vi "XY State Machine Example.vi"() -> ()   [LabVIEW 2019, in "xy_utilities.lvlib"]
uses:
  xy_utilities.lvlib
  subVIs/Derivative (single).vi
  subVIs/Get X and Y (multiple).vi
  subVIs/Add float (multiple).vi
  subVIs/Subtract float (multiple).vi
  subVIs/Multiply float (multiple).vi
  subVIs/Divide float (multiple).vi
  subVIs/Sort (multiple).vi
  subVIs/Swap X and Y (multiple).vi
  subVIs/Reverse (multiple).vi
  subVIs/Subset (multiple).vi
  subVIs/Interpolate (multiple).vi
  subVIs/FFT (multiple).vi
  subVIs/PS (multiple).vi
  subVIs/Resample (multiple).vi
panel:
  in  "Interval Units":enum16{"Points", "Data"}(ring)
  out "Differential":cluster{"X-array":dbl[], "Y-array":dbl[]}(graph)
  out "Processed States":string
  in  "y":dbl format="%#_6p"
  in  "x":dbl format="%#_6p"
  in  "Available States":i32(listbox) caption="States to Process"
  out "FFT":cluster{"f0":dbl, "df":dbl, "magnitude":dbl[]}[](graph)
  in  "Process Queue":string
  in  "PROCESS":bool
  in  "Configure":T1={"X Low"=0.05, "X High"=0.5, "X Step"=0.01, "Fake Point"=0.05} {"Fake Point" format="%#_6p"; "X Step" format="%#_6p"; "X High" format="%#_6p"; "X Low" format="%#_6p"}
  in  "Derivative Type":enum16{"dy/dx vs x", "dx/dy vs y"}(ring)
  in  "Interval":dbl=2.0
  out "Y Arrays":cluster{"Y-array":dbl[]}[](graph)
  out "X Arrays":cluster{"X-array":dbl[]}[](graph)
  in  "STOP":bool
  in  "Subset Slider":cluster{dbl, dbl}(slide)={0.75, 0.25} caption="Horizontal Slider" scale=0.0..1.0
  in  "Subset Method":enum16{"Slider (%)", "X[] min and max"}(ring)
  out "XY Data":cluster{"X-array":dbl[], "Y-array":dbl[]}[](graph)
  # "The \"Process Queue\" is a list of states that will execute when you press the \"PROCESS\" button. (XY: Load and UI: Display Data are added automatically to the beginning and end of the queue.)\n\nTo add states you can either:\n- Type directly into the Process Queue box.\nor:\n- Select a state in the \"Available States\" box that you want to add to the queue. ctl-v in the \"State Queue\" control to add to the queue.\n\nArguments for the various methods are found below"
  # "Arithmetic\n(+ - * /)"
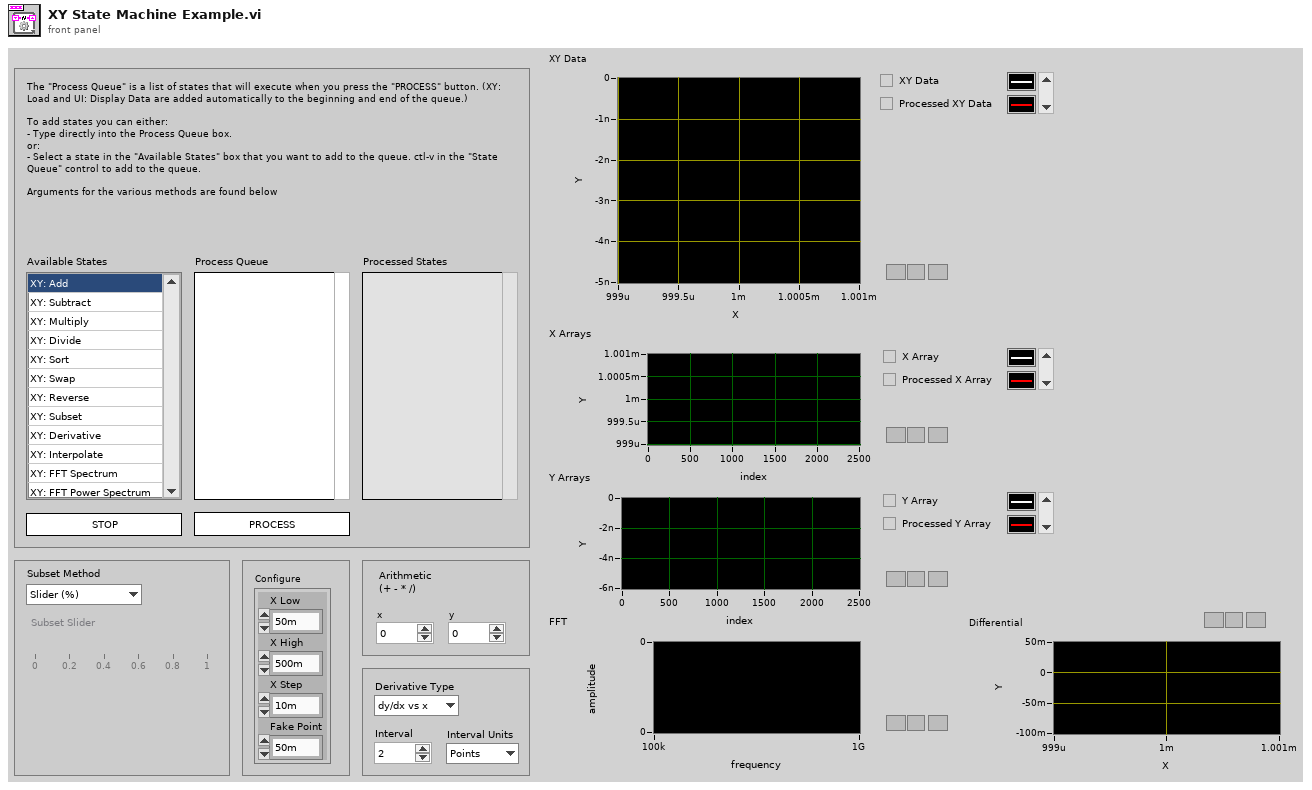
[diagram p1: front panel]
types:
  T1 = cluster{"X Low":dbl, "X High":dbl, "X Step":dbl, "Fake Point":dbl}
  T2 = enum32{"Invalid", "Standard", "Closed", "Hidden", "Minimized", "Maximized"}
  T3 = enum32{"invalid app kind", "Development System", "Run Time System", "Student Edition", "Embedded LabVIEW", "Evaluation", "Custom"}
  T4 = cluster{"Shift":bool, "Ctrl":bool, "Alt":bool, "Cmd":bool, "Opt":bool}
  T5 = cluster{"Core":cluster{"Current VI Reference":refnum<vi>, "Close Panel on Exit?":bool}, "XY Data (unprocessed)":cluster{"Intensity Data":dbl[], "Array":dbl[]}[], "XY Data":cluster{"Intensity Data":dbl[], "Array":dbl[]}[]}
  T6 = cluster{"Current VI Reference":refnum<vi>, "Close Panel on Exit?":bool}
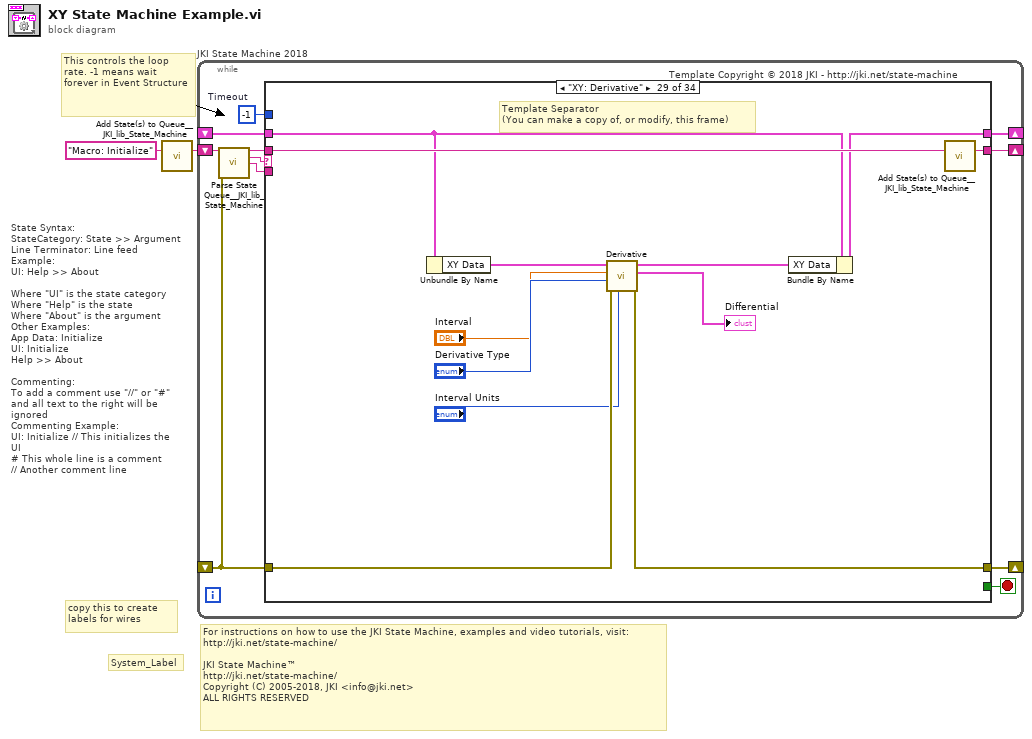
[diagram p0: block diagram]
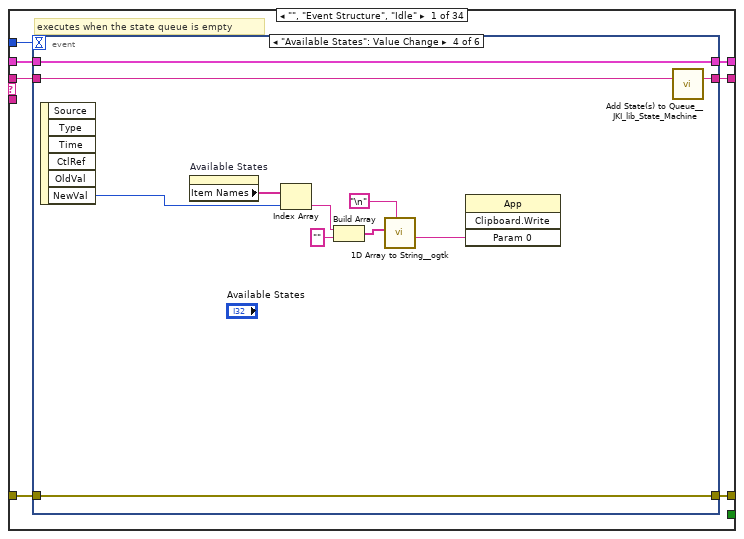
[diagram p2: hidden frame]
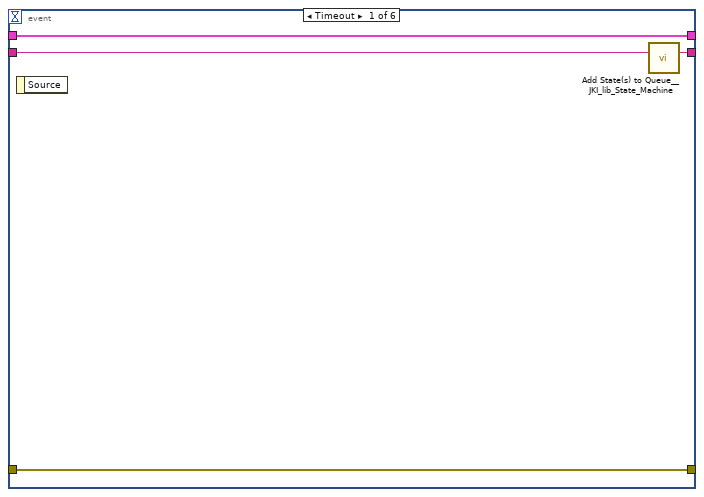
[diagram p3: hidden frame]
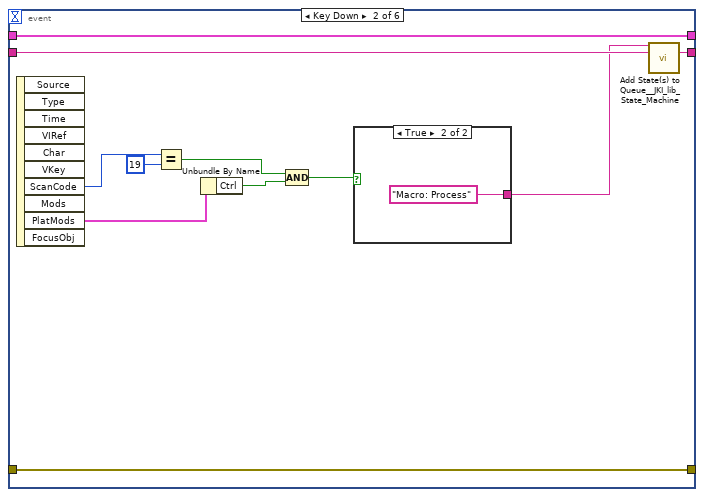
[diagram p4: hidden frame]
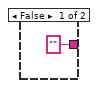
[diagram p5: hidden frame]
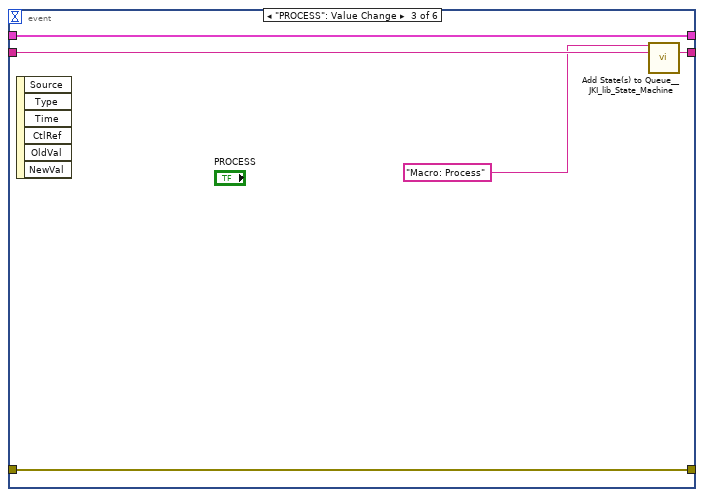
[diagram p6: hidden frame]
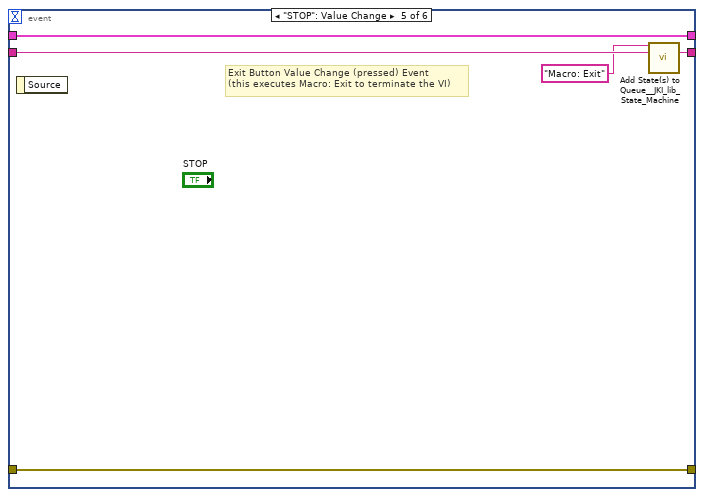
[diagram p7: hidden frame]
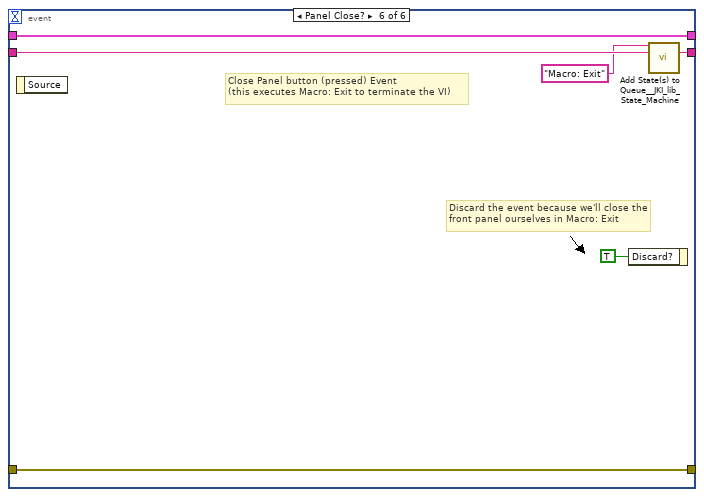
[diagram p8: hidden frame]
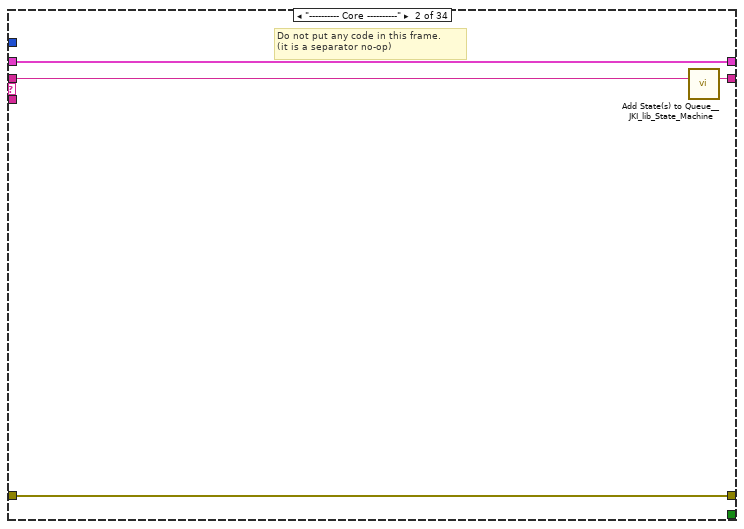
[diagram p9: hidden frame]
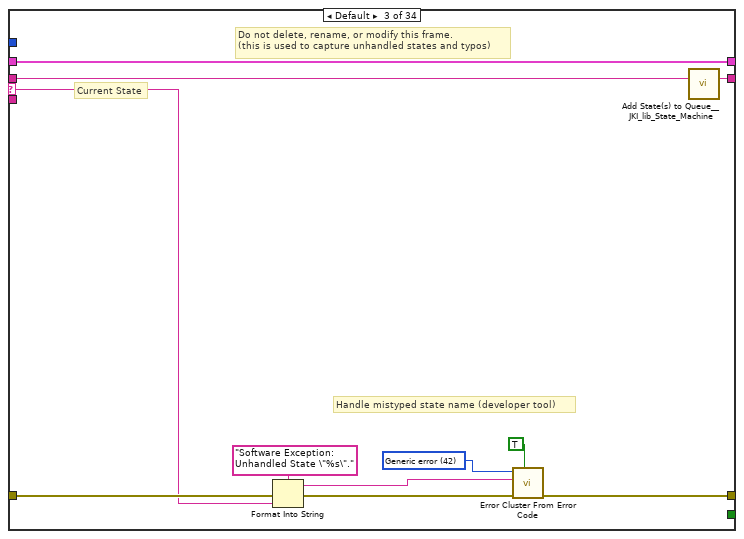
[diagram p10: hidden frame]
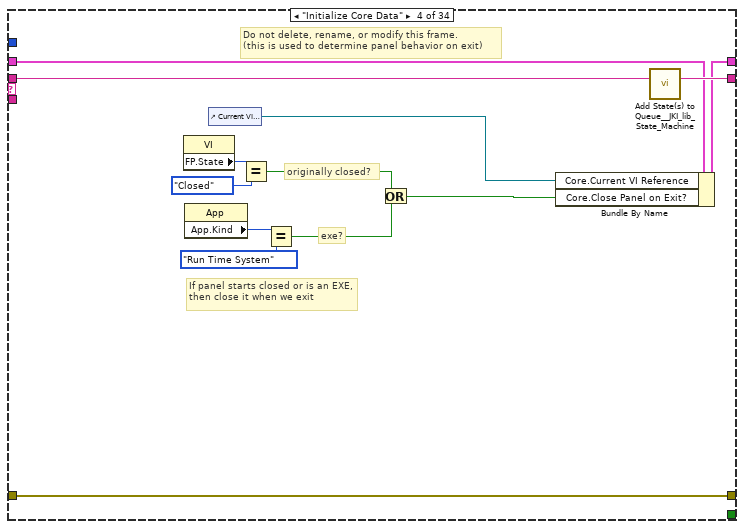
[diagram p11: hidden frame]
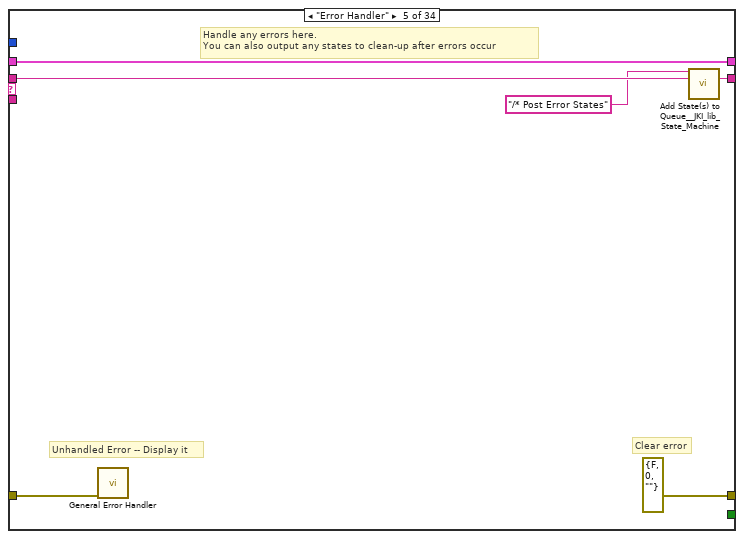
[diagram p12: hidden frame]
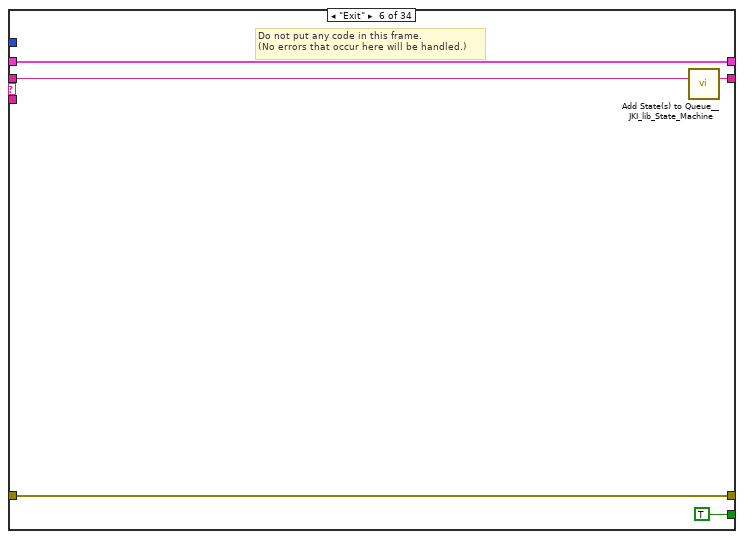
[diagram p13: hidden frame]
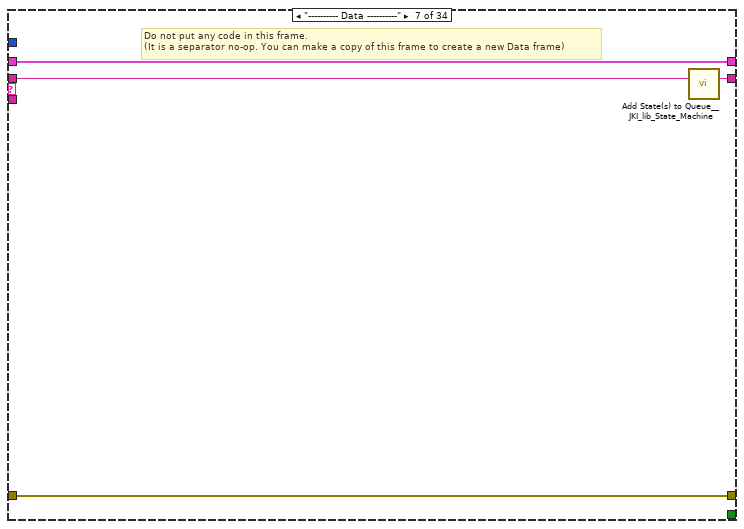
[diagram p14: hidden frame]
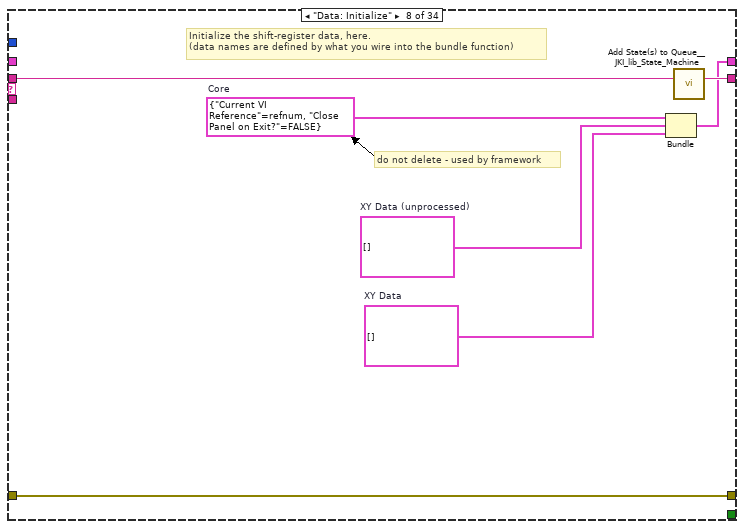
[diagram p15: hidden frame]
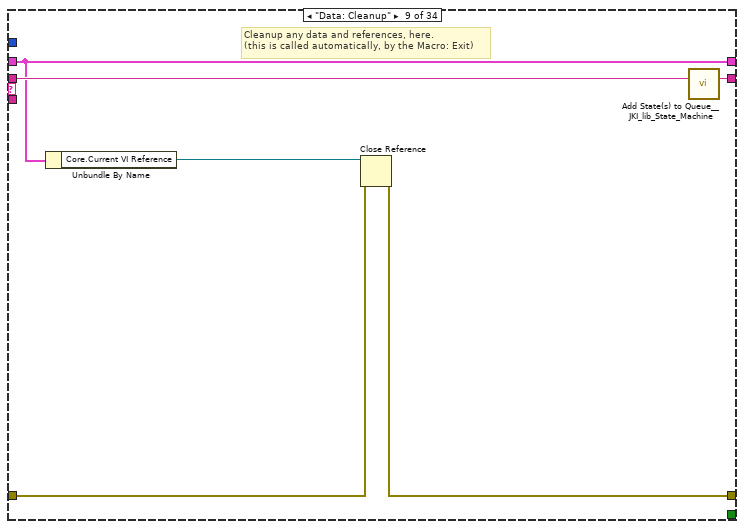
[diagram p16: hidden frame]
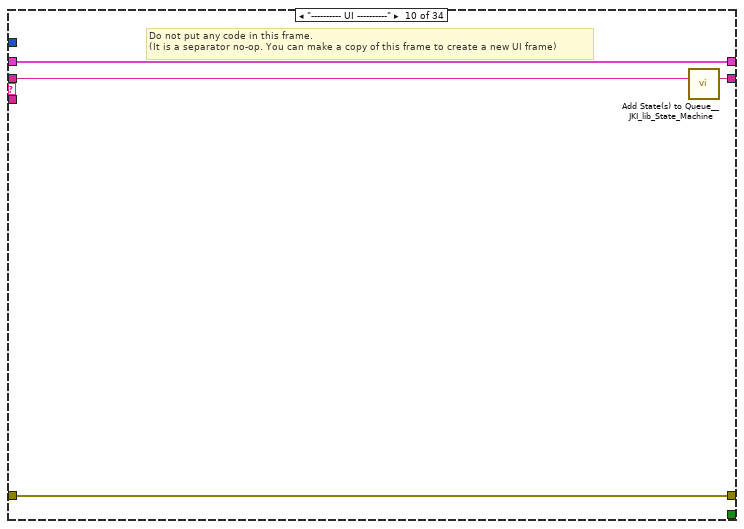
[diagram p17: hidden frame]
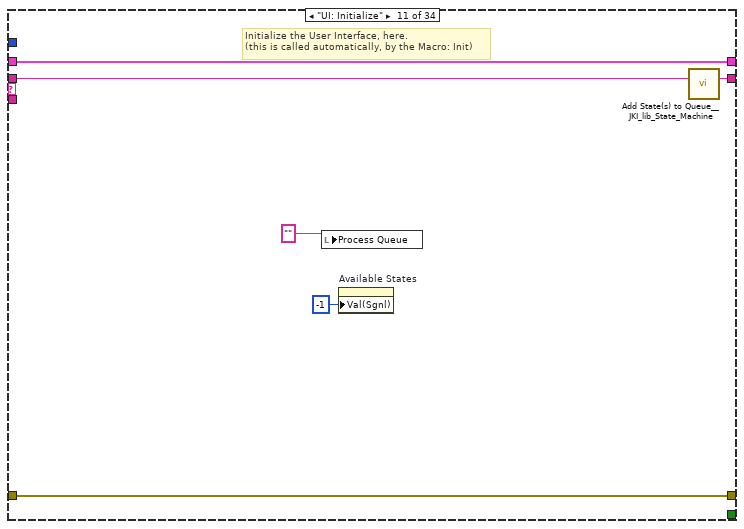
[diagram p18: hidden frame]
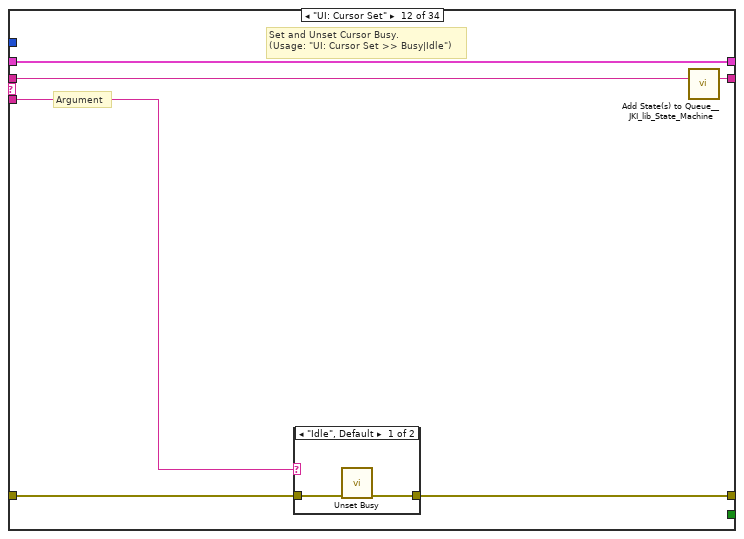
[diagram p19: hidden frame]
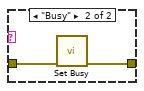
[diagram p20: hidden frame]
diagram:
  # "For instructions on how to use the JKI State Machine, examples and video tutorials, visit:\nhttp://jki.net/state-machine/\n\nJKI State Machine™\nhttp://jki.net/state-machine/\nCopyright (C) 2005-2018, JKI <info@jki.net>\nALL RIGHTS RESERVED"
  # "State Syntax:\nStateCategory: State >> Argument\nLine Terminator: Line feed\nExample:\nUI: Help >> About\n\nWhere \"UI\" is the state category\nWhere \"Help\" is the state\nWhere \"About\" is the argument\nOther Examples:\nApp Data: Initialize\nUI: Initialize\nHelp >> About\n\nCommenting:\nTo add a comment use \"//\" or \"#\" and all text to the right will be ignored\nCommenting Example:\nUI: Initialize // This initializes the UI\n# This whole line is a comment\n// Another comment line"
  # "copy this to create labels for wires"
  # "This controls the loop rate. -1 means wait forever in Event Structure"
  # "System_Label"
  n1 = call <vilib>:"Add State(s) to Queue__JKI_lib_State_Machine.vi"("State(s) in (\"\")"="Macro: Initialize") -> ("States Out"=w2:string)  [unwired: 14 in]
  n2 = while "JKI State Machine 2018" {
    shift-right: [w6] -> _
    shift-left: _ -> [w5]
    shift-right: [w9] -> _
    shift-left: _ -> [w3]
    shift-right: [w8] -> _
    shift-left: w2 -> [w10]
    stop <- w7 stop-if-true
    w4 = -1  # Timeout
    # "Template Copyright © 2018 JKI - http://jki.net/state-machine"
    n3 = call <vilib>:"Parse State Queue__JKI_lib_State_Machine.vi"("State Queue"=w10, "Error In (no error)"=w3) -> ("Remaining States"=w12:string, "Current State"=w13:string, "Arguments"=w11:string)  [unwired: 11 in]
    n4 = case shown="\"XY: Derivative\"" w13 {
      selector: w13 -> [_ _ w69 _ _ _ _ _ _ _ _ _ _ _ _ _ _ _ _ _ _ _ _ _ _ _ _ _ _ _ _ _ _ _]
      tunnel: w12 -> [w20 w68 w73 w92 w98 w103 w107 w114 w120 w124 w130 w136 w147 w223 w227 w232 w242 w250 w258 w264 w274 w284 w294 w304 w312 w320 w328 w338 w350 w359 w368 w377 w385 w393]
      tunnel: w11 -> [_ _ _ _ _ _ _ _ _ _ _ w131 w141 _ _ _ _ _ _ _ _ _ _ _ _ _ _ _ _ _ _ _ _ _]
      tunnel: w5 -> [w18 w65 w71 w85 w95 w101 w104 _ w115 w121 w128 w134 w143 w219 w224 w229 w239 w247 w255 w261 w271 w281 w291 w301 w309 w317 w325 w335 w347 w356 w365 w374 w382 w390]
      tunnel: [w17 w66 w75 w89 errorcluster {"status"=FALSE, "code"=0, "source"=""} ("error out") w100 w105 w111 w116 w122 w127 w132 w144 w216 w225 w230 w240 w248 w251 w262 w267 w277 w287 w297 w305 w313 w321 w331 w343 w352 w361 w371 w378 w386] -> w9
      tunnel: w3 -> [w16 w66 w74 w89 w94 w100 w105 w111 w117 w122 w127 w133 w145 w217 w225 w230 w240 w248 w252 w262 w268 w278 w288 w298 w306 w314 w322 w332 w344 w353 w362 w372 w379 w387]
      tunnel: [w19 w67 w72 w91 w97 w102 w106 w113 w119 w123 w129 w135 w146 w222 w226 w231 w241 w249 w257 w263 w273 w283 w293 w303 w311 w319 w327 w337 w349 w358 w367 w376 w384 w392] -> w8
      tunnel: [_ _ _ _ _ TRUE _ _ _ _ _ _ _ _ _ _ _ _ _ _ _ _ _ _ _ _ _ _ _ _ _ _ _ _] -> w7
      tunnel: [w15 w65 w71 w90 w95 w101 w104 w112 w115 w121 w128 w134 w143 w219 w224 w229 w239 w247 w254 w260 w270 w280 w290 w300 w308 w316 w324 w334 w346 w355 w364 w373 w381 w389] -> w6
      tunnel: w4 -> [w14 _ _ _ _ _ _ _ _ _ _ _ _ _ _ _ _ _ _ _ _ _ _ _ _ _ _ _ _ _ _ _ _ _]
      frame "", "Event Structure", "Idle" {
        # "executes when the state queue is empty"
        n5 = event shown="[3] \"Available States\": Value Change" {
          selector: _ -> [_ _ _ _ _ _]
          dyn-events: _ -> [_ _ _ _ _ _]
          timeout: w14 -> [_ _ _ _ _ _]
          tunnel: w20 -> [w24 w35 w42 w53 w58 w64]
          tunnel: [w23 w34 w41 w52 w57 w63] -> w19
          tunnel: w18 -> [w21 w32 w39 w50 w55 w61]
          tunnel: [w22 w33 w40 w51 w56 w62] -> w17
          tunnel: w16 -> [w22 w33 w40 w51 w56 w62]
          tunnel: [w21 w32 w39 w50 w55 w61] -> w15
          event Timeout {
            n6 = event-data() -> ()  [unwired: 1 in, 1 out]
            n7 = call <vilib>:"Add State(s) to Queue__JKI_lib_State_Machine.vi"("State(s) in (\"\")"=w24) -> ("States Out"=w23:string)  [unwired: 14 in]
          }
          event Key Down {
            n8 = event-data() -> ("ScanCode"=w25:i16, "PlatMods"=w26:T4)  [unwired: 1 in, 8 out]
            n9 = Equal?(x=w25, y=i16 19) -> (x = y?=w28:bool)
            n10 = Unbundle By Name(w26) -> ("Ctrl"=w29:bool)
            n11 = Compound Arithmetic op=AND(w28, w29) -> (w27:bool)
            n12 = case shown="True" w27 {
              tunnel: ["" ("State(s) in Front (\"\")") "Macro: Process" ("State(s) in Front (\"\")")] -> w30
              frame False {
              }
              frame True {
              }
            }
            n13 = call <vilib>:"Add State(s) to Queue__JKI_lib_State_Machine.vi"("State(s) in Front (\"\")"=w30, "State(s) in (\"\")"=w35) -> ("States Out"=w34:string)  [unwired: 13 in]
          }
          event "PROCESS": Value Change {
            n14 = event-data() -> ()  [unwired: 1 in, 6 out]
            n15 = call <vilib>:"Add State(s) to Queue__JKI_lib_State_Machine.vi"("State(s) in Front (\"\")"="Macro: Process" ("State(s) in Front (\"\")"), "State(s) in (\"\")"=w42) -> ("States Out"=w41:string)  [unwired: 13 in]
          }
          event "Available States": Value Change {
            n16 = event-data() -> ("NewVal"=w44:i32)  [unwired: 1 in, 5 out]
            n17 = property on="Available States" class="LstBox (strict)"() -> ("Item Names"=w45:string[])  [unwired: 2 in, 2 out]
            n18 = Index Array(array=w45, index=w44) -> (element=w49:string)
            n19 = Build Array(w49, "" ("element")) -> (w46:string[])
            n20 = call "1D Array to String__ogtk.vi"("delimiter (Tab)"="\n", "Array of Strings"=w46) -> ("delimited string"=w47:string)  [unwired: 9 in]
            n21 = invoke class="App" method="Clipboard.Write"("Param 0"=w47) -> ()  [unwired: 3 in, 4 out]
            n22 = call <vilib>:"Add State(s) to Queue__JKI_lib_State_Machine.vi"("State(s) in (\"\")"=w53) -> ("States Out"=w52:string)  [unwired: 14 in]
          }
          event "STOP": Value Change {
            # "Exit Button Value Change (pressed) Event\n(this executes Macro: Exit to terminate the VI)"
            n23 = event-data() -> ()  [unwired: 1 in, 1 out]
            n24 = call <vilib>:"Add State(s) to Queue__JKI_lib_State_Machine.vi"("State(s) in Front (\"\")"="Macro: Exit", "State(s) in (\"\")"=w58) -> ("States Out"=w57:string)  [unwired: 13 in]
          }
          event Panel Close? {
            # "Discard the event because we'll close the front panel ourselves in Macro: Exit"
            # "Close Panel button (pressed) Event\n(this executes Macro: Exit to terminate the VI)"
            n25 = event-data() -> ()  [unwired: 1 in, 1 out]
            n26 = event-data("Discard?"=TRUE) -> ()  [unwired: 1 in, 1 out]
            n27 = call <vilib>:"Add State(s) to Queue__JKI_lib_State_Machine.vi"("State(s) in Front (\"\")"="Macro: Exit", "State(s) in (\"\")"=w64) -> ("States Out"=w63:string)  [unwired: 13 in]
          }
        }
      }
      frame "---------- Core ----------" {
        # "Do not put any code in this frame.\n(it is a separator no-op)"
        n28 = call <vilib>:"Add State(s) to Queue__JKI_lib_State_Machine.vi"("State(s) in (\"\")"=w68) -> ("States Out"=w67:string)  [unwired: 14 in]
      }
      frame Default {
        w78 = 42 items=["No error", "Argument error", "Memory is full", "Out of zone", "End of file", "File already open", "Generic file I/O error", "File not found", "File permission error", "Disk is full", "Duplicate path", "Too many files open", "System feature not enabled", "Resource file not found", "Cannot add resource", "Resource not found", "Image not found", "Image memory error", "Pen does not exist", "Config type invalid", "Config token not found", "Config parse error", "Config memory error", "Bad external code format", "Bad external code offset", "External code not present", "Null window", "Destroy window error", "Null menu", "Print aborted", "Bad print record", "Print driver error", "Windows error during printing", "Memory error during printing", "Print dialog error", "Generic print error", "Invalid device refnum", "Device not found", "Device parameter error", "Device unit error", "Cannot open device", "Device call aborted", "Generic error", "Cancelled by user", "Object ID too low", "Object ID too high", "Object not in heap", "Unknown heap", "Unknown object (invalid DefProc)", "Unknown object (DefProc not in table)", "Message out of range", "Invalid (null) method", "Unknown message", "Manager call not supported", "Bad address", "Network operation in progress", "Network operation timed out", "Connection is busy", "Network attribute not supported", "Network error", "Address in use", "System out of memory", "Connection aborted", "Connection refused", "Not connected", "Already connected", "Connection closed", "Initialization error (interapplication manager)", "Bad occurrence", "Wait on unbound occurrence handler", "Occurrence queue overflow", "Datalog type conflict", "Unused", "Unrecognized type (interapplication manager)", "Memory corrupt", "Failed to make temporary DLL", "Old CIN version", "Drag socket not found", "Failed to load drop-object", "Failed to register OLE object", "Failed to release OLE object", "Format specifier type mismatch", "Unknown format specifier", "Too few format specifiers", "Too many format specifiers", "Scan failed", "Newer CIN version", "Error converting to variant", "Runtime menu error", "Password tampered", "Variant attribute not found", "Incompatible variant data type", "Event data is not available", "Event Store is not present", "Occurrence is not found", "Event Queue is not created", "Event info is not available", "Refnum passed is NULL", "Error retrieving Class GUID", "Error retrieving CoClass GUID", "Error retrieving TypeLib GUID.", "Bad built application magic bytes.", "Specific driver is different from the specific driver associated with the Logical Name.", "There is no session opened to the class driver.", "Max Error", "MAX - Error with config objects", "MAX - Error loading configuration", "MAX - Group not supported"]
        # "Current State"
        # "Do not delete, rename, or modify this frame.\n(this is used to capture unhandled states and typos)"
        # "Handle mistyped state name (developer tool)"
        n29 = Format Into String(format string="Software Exception: Unhandled State \"%s\"." ("message"), error in=w74, w69) -> (resulting string=w77:string, error out=w76:errorcluster)  [unwired: 1 in]
        n30 = call <vilib>:"Error Cluster From Error Code.vi"("show call chain? (False)"=TRUE, "error in (no error)"=w76, "error message (\"\")"=w77, "error code (0)"=w78) -> ("error out"=w75:errorcluster)  [unwired: 5 in]
        n31 = call <vilib>:"Add State(s) to Queue__JKI_lib_State_Machine.vi"("State(s) in (\"\")"=w73) -> ("States Out"=w72:string)  [unwired: 14 in]
      }
      frame "Initialize Core Data" {
        # "Do not delete, rename, or modify this frame.\n(this is used to determine panel behavior on exit)"
        # "originally closed?"
        # "exe?"
        # "If panel starts closed or is an EXE, then close it when we exit"
        n32 = property class="VI"() -> ("FP.State"=w82:T2)  [unwired: 2 in, 2 out]
        n33 = property class="App"() -> ("App.Kind"=w88:T3)  [unwired: 2 in, 2 out]
        n34 = control-ref of="Current VI Reference"() -> (w83:refnum<vi>)
        n35 = Equal?(x=w82, y=T2."Closed" ("Front Panel Window:State")) -> (x = y?=w80:bool)
        n36 = Equal?(x=w88, y=T3."Run Time System" ("Application:Kind")) -> (x = y?=w86:bool)
        n37 = Or(x=w80, y=w86) -> (x .or. y?=w84:bool)
        n38 = Bundle By Name(cluster=w85, "Core.Current VI Reference"=w83, "Core.Close Panel on Exit?"=w84) -> (w90:T5)
        n39 = call <vilib>:"Add State(s) to Queue__JKI_lib_State_Machine.vi"("State(s) in (\"\")"=w92) -> ("States Out"=w91:string)  [unwired: 14 in]
      }
      frame "Error Handler" {
        # "Unhandled Error -- Display it"
        # "Handle any errors here.\nYou can also output any states to clean-up after errors occur"
        # "Clear error"
        n40 = call <vilib>:"General Error Handler.vi"("error in (no error)"=w94) -> ()  [unwired: 10 in, 5 out]
        n41 = call <vilib>:"Add State(s) to Queue__JKI_lib_State_Machine.vi"("State(s) in Front (\"\")"="/* Post Error States", "State(s) in (\"\")"=w98) -> ("States Out"=w97:string)  [unwired: 13 in]
      }
      frame "Exit" {
        # "Do not put any code in this frame.\n(No errors that occur here will be handled.)"
        n42 = call <vilib>:"Add State(s) to Queue__JKI_lib_State_Machine.vi"("State(s) in (\"\")"=w103) -> ("States Out"=w102:string)  [unwired: 14 in]
      }
      frame "---------- Data ----------" {
        # "Do not put any code in this frame.\n(It is a separator no-op. You can make a copy of this frame to create a new Data frame)"
        n43 = call <vilib>:"Add State(s) to Queue__JKI_lib_State_Machine.vi"("State(s) in (\"\")"=w107) -> ("States Out"=w106:string)  [unwired: 14 in]
      }
      frame "Data: Initialize" {
        w108 = cluster{"Intensity Data":dbl[], "Array":dbl[]}[] []  # XY Data
        w109 = cluster{"Intensity Data":dbl[], "Array":dbl[]}[] []  # XY Data (unprocessed)
        w110 = T6 {"Current VI Reference"=refnum, "Close Panel on Exit?"=FALSE}  # Core
        # "do not delete - used by framework"
        # "Initialize the shift-register data, here.\n(data names are defined by what you wire into the bundle function)"
        n44 = Bundle("Core"=w110, "XY Data (unprocessed)"=w109, "XY Data"=w108) -> (w112:T5)  [unwired: 1 in]
        n45 = call <vilib>:"Add State(s) to Queue__JKI_lib_State_Machine.vi"("State(s) in (\"\")"=w114) -> ("States Out"=w113:string)  [unwired: 14 in]
      }
      frame "Data: Cleanup" {
        # "Cleanup any data and references, here.\n(this is called automatically, by the Macro: Exit)"
        n46 = Unbundle By Name(w115) -> ("Core.Current VI Reference"=w118:refnum<vi>)
        n47 = Close Reference(reference=w118, error in (no error)=w117) -> (error out=w116:errorcluster)
        n48 = call <vilib>:"Add State(s) to Queue__JKI_lib_State_Machine.vi"("State(s) in (\"\")"=w120) -> ("States Out"=w119:string)  [unwired: 14 in]
      }
      frame "---------- UI ----------" {
        # "Do not put any code in this frame.\n(It is a separator no-op. You can make a copy of this frame to create a new UI frame)"
        n49 = call <vilib>:"Add State(s) to Queue__JKI_lib_State_Machine.vi"("State(s) in (\"\")"=w124) -> ("States Out"=w123:string)  [unwired: 14 in]
      }
      frame "UI: Initialize" {
        # "Initialize the User Interface, here.\n(this is called automatically, by the Macro: Init)"
        n50 = local write "Process Queue"("" ("Process States")) -> ()
        n51 = property on="Available States" class="LstBox (strict)"("Val(Sgnl)"=-1 ("Value (Signaling)")) -> ()  [unwired: 2 in, 2 out]
        n52 = call <vilib>:"Add State(s) to Queue__JKI_lib_State_Machine.vi"("State(s) in (\"\")"=w130) -> ("States Out"=w129:string)  [unwired: 14 in]
      }
      frame "UI: Cursor Set" {
        # "Argument"
        # "Set and Unset Cursor Busy.\n(Usage: \"UI: Cursor Set >> Busy|Idle\")"
        n53 = case shown="\"Idle\", Default" w131 {
          tunnel: w133 -> [w138 w140]
          tunnel: [w137 w139] -> w132
          frame "Idle", Default {
            n54 = call <vilib>:"Unset Busy.vi"("error in (no error)"=w138) -> ("error out"=w137:errorcluster)  [unwired: 10 in]
          }
          frame "Busy" {
            n55 = call <vilib>:"Set Busy.vi"("error in (no error)"=w140) -> ("error out"=w139:errorcluster)  [unwired: 9 in, 1 out]
          }
        }
        n56 = call <vilib>:"Add State(s) to Queue__JKI_lib_State_Machine.vi"("State(s) in (\"\")"=w136) -> ("States Out"=w135:string)  [unwired: 14 in]
      }
      frame "UI: Front Panel State" {
        # "Argument"
        # "Set Front Panel Open or Closed\n(Usage: \"UI: Front Panel State >> Open|Close\")"
        n57 = Unbundle By Name(w143) -> ("Core.Current VI Reference"=w142:refnum<vi>)
        n58 = case shown="\"Maximize\", \"Maximized\"" w141 {
          tunnel: w145 -> [w153 w168 w179 w192 w205]
          tunnel: [w155 w169 w181 w194 w207] -> w144
          tunnel: w142 -> [w154 w166 w180 w193 w206]
          frame "Open", "Standard", Default {
            w148 = T2."Standard" ("State")
            n59 = property class="VI"(reference=w154, error in=w153) -> (reference out=w151:refnum<vi>, error out=w152:errorcluster, "FP.State"=w150:T2)
            n60 = Not Equal?(x=w150, y=w148) -> (x != y?=w149:bool)
            n61 = case shown="True" w149 {
              tunnel: [w159 w161] -> w155
              tunnel: w152 -> [w158 w161]
              tunnel: w151 -> [w157 _]
              tunnel: w148 -> [w156 _]
              frame True {
                n62 = invoke class="VI" method="FP.Open"(reference=w157, error in=w158, "Activate"=TRUE, "State"=w156) -> (error out=w159:errorcluster)  [unwired: 1 in, 4 out]
              }
              frame False {
              }
            }
          }
          frame "Close", "Closed" {
            n63 = property class="VI"(reference=w166, error in=w168) -> (reference out=w165:refnum<vi>, error out=w167:errorcluster, "FP.State"=w163:T2)
            n64 = Not Equal?(x=w163, y=T2."Closed" ("Front Panel Window:State")) -> (x != y?=w162:bool)
            n65 = case shown="True" w162 {
              tunnel: [w170 w173] -> w169
              tunnel: w167 -> [w170 w172]
              tunnel: w165 -> [_ w171]
              frame False {
              }
              frame True {
                n66 = invoke class="VI" method="FP.Close"(reference=w171, error in=w172) -> (error out=w173:errorcluster)  [unwired: 1 in, 2 out]
              }
            }
          }
          frame "Hidden", "Hide" {
            w174 = T2."Hidden" ("State")
            n67 = property class="VI"(reference=w180, error in=w179) -> (reference out=w177:refnum<vi>, error out=w178:errorcluster, "FP.State"=w176:T2)
            n68 = Not Equal?(x=w176, y=w174) -> (x != y?=w175:bool)
            n69 = case shown="True" w175 {
              tunnel: [w185 w186] -> w181
              tunnel: w178 -> [w184 w186]
              tunnel: w177 -> [w183 _]
              tunnel: w174 -> [w182 _]
              frame True {
                n70 = invoke class="VI" method="FP.Open"(reference=w183, error in=w184, "State"=w182) -> (error out=w185:errorcluster)  [unwired: 2 in, 4 out]
              }
              frame False {
              }
            }
          }
          frame "Minimize", "Minimized" {
            w187 = T2."Minimized" ("State")
            n71 = property class="VI"(reference=w193, error in=w192) -> (reference out=w190:refnum<vi>, error out=w191:errorcluster, "FP.State"=w189:T2)
            n72 = Not Equal?(x=w189, y=w187) -> (x != y?=w188:bool)
            n73 = case shown="True" w188 {
              tunnel: [w198 w199] -> w194
              tunnel: w191 -> [w197 w199]
              tunnel: w190 -> [w196 _]
              tunnel: w187 -> [w195 _]
              frame True {
                n74 = invoke class="VI" method="FP.Open"(reference=w196, error in=w197, "State"=w195) -> (error out=w198:errorcluster)  [unwired: 2 in, 4 out]
              }
              frame False {
              }
            }
          }
          frame "Maximize", "Maximized" {
            w200 = T2."Maximized" ("State")
            n75 = property class="VI"(reference=w206, error in=w205) -> (reference out=w203:refnum<vi>, error out=w204:errorcluster, "FP.State"=w202:T2)
            n76 = Not Equal?(x=w202, y=w200) -> (x != y?=w201:bool)
            n77 = case shown="True" w201 {
              tunnel: [w211 w212] -> w207
              tunnel: w204 -> [w210 w212]
              tunnel: w203 -> [w209 _]
              tunnel: w200 -> [w208 _]
              frame True {
                n78 = invoke class="VI" method="FP.Open"(reference=w209, error in=w210, "State"=w208) -> (error out=w211:errorcluster)  [unwired: 2 in, 4 out]
              }
              frame False {
              }
            }
          }
        }
        n79 = call <vilib>:"Add State(s) to Queue__JKI_lib_State_Machine.vi"("State(s) in (\"\")"=w147) -> ("States Out"=w146:string)  [unwired: 14 in]
      }
      frame "UI: Display Data" {
        # "Do not put any code in this frame.\n(It is a separator no-op. You can make a copy of this frame to create a new UI frame)"
        n80 = Unbundle By Name(w219) -> ("XY Data (unprocessed)"=w221:cluster{"Intensity Data":dbl[], "Array":dbl[]}[], "XY Data"=w220:cluster{"Intensity Data":dbl[], "Array":dbl[]}[])
        n81 = Build Array (concatenate)(w221, w220) -> (w215:cluster{"Intensity Data":dbl[], "Array":dbl[]}[])
        n82 = call-poly "Get X and Y.vi"("error in (no error)"=w217, "XY-data"=w215) -> ("error out"=w216:errorcluster, "Y-Arrays"=→"Y Arrays":cluster{"Y-array":dbl[]}[], "X-Arrays"=→"X Arrays":cluster{"X-array":dbl[]}[], "XY-data out"=→"XY Data":cluster{"X-array":dbl[], "Y-array":dbl[]}[])  [unwired: 6 in]
        n83 = call <vilib>:"Add State(s) to Queue__JKI_lib_State_Machine.vi"("State(s) in (\"\")"=w223) -> ("States Out"=w222:string)  [unwired: 14 in]
      }
      frame "---------- Macro ----------" {
        # "Do not put any code in this frame.\n(It is a separator no-op. You can make a copy of this frame to create a new Macro frame)"
        n84 = call <vilib>:"Add State(s) to Queue__JKI_lib_State_Machine.vi"("State(s) in (\"\")"=w227) -> ("States Out"=w226:string)  [unwired: 14 in]
      }
      frame "Macro: Initialize" {
        w228 = "Data: Initialize\nInitialize Core Data\nUI: Initialize\nUI: Front Panel State >> Open"  # Data: Initialize Initialize Core Data UI: Initialize UI: Front Panel State >> Open
        # "Initialization Macro\n(This is called once, when the VI starts)"
        n85 = call <vilib>:"Add State(s) to Queue__JKI_lib_State_Machine.vi"("State(s) in Front (\"\")"=w228, "State(s) in (\"\")"=w232) -> ("States Out"=w231:string)  [unwired: 13 in]
      }
      frame "Macro: Exit" {
        # "Exit Macro\n(This is called once, when the VI exits)"
        n86 = Unbundle By Name(w239) -> ("Core.Close Panel on Exit?"=w238:bool)
        n87 = Select(t="UI: Front Panel State >> Close", s=w238, f="") -> (s? t:f=w235:string)
        n88 = call <vilib>:"Add State(s) to Queue__JKI_lib_State_Machine.vi"("State(s) in (\"\")"=w235, "State(s) at Back (\"\")"="Data: Cleanup\nExit") -> ("States Out"=w233:string)  [unwired: 13 in]
        n89 = call <vilib>:"Add State(s) to Queue__JKI_lib_State_Machine.vi"("State(s) in Front (\"\")"=w233, "State(s) in (\"\")"=w242) -> ("States Out"=w241:string)  [unwired: 13 in]
      }
      frame "Macro: Process" {
        # "XY: Add\nXY: Subtract\nXY: Multiply\nXY: Divide\nXY: Sort\nXY: Swap\nXY: Reverse\nXY: Subset\nXY: Derivative\nXY: Interpolate\nXY: FFT Spectrum\nXY: FFT Power Spectrum"
        # "Do not put any code in this frame.\n(It is a separator no-op. You can make a copy of this frame to create a new Macro frame)"
        n90 = call <vilib>:"Add State(s) to Queue__JKI_lib_State_Machine.vi"("State(s) in Front (\"\")"="XY: Load" ("State(s) in Front (\"\")"), "State(s) in (\"\")"="Process Queue", "State(s) at Back (\"\")"="UI: Display Data" ("State(s) in Front (\"\")")) -> ("States Out"=w243:string)  [unwired: 12 in]
        "Processed States" <- w243
        n91 = call <vilib>:"Add State(s) to Queue__JKI_lib_State_Machine.vi"("State(s) in Front (\"\")"=w243, "State(s) in (\"\")"=w250) -> ("States Out"=w249:string)  [unwired: 13 in]
      }
      frame "---------- XY ----------" {
        # "Template Separator\n(You can make a copy of, or modify, this frame)"
        n92 = Unbundle By Name(w255) -> ("XY Data"=w256:cluster{"Intensity Data":dbl[], "Array":dbl[]}[])
        n93 = call-poly "Add.vi"("error in (no error)"=w252, "XY-data"=w256) -> ("error out"=w251:errorcluster, "XY-data out"=w253:cluster{"X-array":dbl[], "Y-array":dbl[]}[])  [unwired: 8 in]
        n94 = Bundle By Name(cluster=w255, "XY Data"=w253) -> (w254:T5)
        n95 = call <vilib>:"Add State(s) to Queue__JKI_lib_State_Machine.vi"("State(s) in (\"\")"=w258) -> ("States Out"=w257:string)  [unwired: 14 in]
      }
      frame "XY: Load" {
        w259 = cluster{"Intensity Data":dbl[], "Array":dbl[]}[] [{"Intensity Data"=array[2480 elements], "Array"=array[2480 elements]}] ("XY Data 2")
        # "Template Separator\n(You can make a copy of, or modify, this frame)"
        n96 = Unbundle By Name(w261) -> ()  [unwired: 1 out]
        n97 = Bundle By Name(cluster=w261, "XY Data"=w259, "XY Data (unprocessed)"=w259) -> (w260:T5)
        n98 = call <vilib>:"Add State(s) to Queue__JKI_lib_State_Machine.vi"("State(s) in (\"\")"=w264) -> ("States Out"=w263:string)  [unwired: 14 in]
      }
      frame "XY: Add" {
        # "Template Separator\n(You can make a copy of, or modify, this frame)"
        n99 = Unbundle By Name(w271) -> ("XY Data"=w272:cluster{"Intensity Data":dbl[], "Array":dbl[]}[])
        n100 = call-poly "Add.vi"("error in (no error)"=w268, "y (0)"="y", "x (0)"="x", "XY-data"=w272) -> ("error out"=w267:errorcluster, "XY-data out"=w269:cluster{"X-array":dbl[], "Y-array":dbl[]}[])  [unwired: 6 in]
        n101 = Bundle By Name(cluster=w271, "XY Data"=w269) -> (w270:T5)
        n102 = call <vilib>:"Add State(s) to Queue__JKI_lib_State_Machine.vi"("State(s) in (\"\")"=w274) -> ("States Out"=w273:string)  [unwired: 14 in]
      }
      frame "XY: Subtract" {
        # "Template Separator\n(You can make a copy of, or modify, this frame)"
        n103 = Unbundle By Name(w281) -> ("XY Data"=w282:cluster{"Intensity Data":dbl[], "Array":dbl[]}[])
        n104 = local read "x"() -> (w275:dbl)
        n105 = local read "y"() -> (w276:dbl)
        n106 = call-poly "Subtract.vi"("error in (no error)"=w278, "y (0)"=w276, "x (0)"=w275, "XY-data"=w282) -> ("error out"=w277:errorcluster, "XY-data out"=w279:cluster{"X-array":dbl[], "Y-array":dbl[]}[])  [unwired: 6 in]
        n107 = Bundle By Name(cluster=w281, "XY Data"=w279) -> (w280:T5)
        n108 = call <vilib>:"Add State(s) to Queue__JKI_lib_State_Machine.vi"("State(s) in (\"\")"=w284) -> ("States Out"=w283:string)  [unwired: 14 in]
      }
      frame "XY: Multiply" {
        # "Template Separator\n(You can make a copy of, or modify, this frame)"
        n109 = Unbundle By Name(w291) -> ("XY Data"=w292:cluster{"Intensity Data":dbl[], "Array":dbl[]}[])
        n110 = local read "x"() -> (w286:dbl)
        n111 = local read "y"() -> (w285:dbl)
        n112 = call-poly "Multiply.vi"("error in (no error)"=w288, "y (1)"=w285, "x (1)"=w286, "XY-data"=w292) -> ("error out"=w287:errorcluster, "XY-data out"=w289:cluster{"X-array":dbl[], "Y-array":dbl[]}[])  [unwired: 6 in]
        n113 = Bundle By Name(cluster=w291, "XY Data"=w289) -> (w290:T5)
        n114 = call <vilib>:"Add State(s) to Queue__JKI_lib_State_Machine.vi"("State(s) in (\"\")"=w294) -> ("States Out"=w293:string)  [unwired: 14 in]
      }
      frame "XY: Divide" {
        # "Template Separator\n(You can make a copy of, or modify, this frame)"
        n115 = Unbundle By Name(w301) -> ("XY Data"=w302:cluster{"Intensity Data":dbl[], "Array":dbl[]}[])
        n116 = local read "x"() -> (w296:dbl)
        n117 = local read "y"() -> (w295:dbl)
        n118 = call-poly "Divide.vi"("error in (no error)"=w298, "y (1)"=w295, "x (1)"=w296, "XY-data"=w302) -> ("error out"=w297:errorcluster, "XY-data out"=w299:cluster{"X-array":dbl[], "Y-array":dbl[]}[])  [unwired: 6 in]
        n119 = Bundle By Name(cluster=w301, "XY Data"=w299) -> (w300:T5)
        n120 = call <vilib>:"Add State(s) to Queue__JKI_lib_State_Machine.vi"("State(s) in (\"\")"=w304) -> ("States Out"=w303:string)  [unwired: 14 in]
      }
      frame "XY: Sort" {
        # "Template Separator\n(You can make a copy of, or modify, this frame)"
        n121 = Unbundle By Name(w309) -> ("XY Data"=w310:cluster{"Intensity Data":dbl[], "Array":dbl[]}[])
        n122 = call-poly "Sort.vi"("error in (no error)"=w306, "XY-data"=w310) -> ("error out"=w305:errorcluster, "Sorted XY-data out"=w307:cluster{"X-array":dbl[], "Y-array":dbl[]}[])  [unwired: 8 in]
        n123 = Bundle By Name(cluster=w309, "XY Data"=w307) -> (w308:T5)
        n124 = call <vilib>:"Add State(s) to Queue__JKI_lib_State_Machine.vi"("State(s) in (\"\")"=w312) -> ("States Out"=w311:string)  [unwired: 14 in]
      }
      frame "XY: Swap" {
        # "Template Separator\n(You can make a copy of, or modify, this frame)"
        n125 = Unbundle By Name(w317) -> ("XY Data"=w318:cluster{"Intensity Data":dbl[], "Array":dbl[]}[])
        n126 = call-poly "Swap X and Y.vi"("error in (no error)"=w314, "XY-data"=w318) -> ("error out"=w313:errorcluster, "XY-data out"=w315:cluster{"X-array":dbl[], "Y-array":dbl[]}[])  [unwired: 8 in]
        n127 = Bundle By Name(cluster=w317, "XY Data"=w315) -> (w316:T5)
        n128 = call <vilib>:"Add State(s) to Queue__JKI_lib_State_Machine.vi"("State(s) in (\"\")"=w320) -> ("States Out"=w319:string)  [unwired: 14 in]
      }
      frame "XY: Reverse" {
        # "Template Separator\n(You can make a copy of, or modify, this frame)"
        n129 = Unbundle By Name(w325) -> ("XY Data"=w326:cluster{"Intensity Data":dbl[], "Array":dbl[]}[])
        n130 = call-poly "Reverse.vi"("error in (no error)"=w322, "XY-data"=w326) -> ("error out"=w321:errorcluster, "Reversed XY-data out"=w323:cluster{"X-array":dbl[], "Y-array":dbl[]}[])  [unwired: 8 in]
        n131 = Bundle By Name(cluster=w325, "XY Data"=w323) -> (w324:T5)
        n132 = call <vilib>:"Add State(s) to Queue__JKI_lib_State_Machine.vi"("State(s) in (\"\")"=w328) -> ("States Out"=w327:string)  [unwired: 14 in]
      }
      frame "XY: Subset" {
        # "Template Separator\n(You can make a copy of, or modify, this frame)"
        n133 = Unbundle By Name(w335) -> ("XY Data"=w336:cluster{"Intensity Data":dbl[], "Array":dbl[]}[])
        n134 = call-poly "Subset.vi"("error in (no error)"=w332, "Subset Method"="Subset Method", "Subset Slider"="Subset Slider", "XY-data"=w336) -> ("error out"=w331:errorcluster, "Subset XY-data out"=w333:cluster{"X-array":dbl[], "Y-array":dbl[]}[])  [unwired: 6 in]
        n135 = Bundle By Name(cluster=w335, "XY Data"=w333) -> (w334:T5)
        n136 = call <vilib>:"Add State(s) to Queue__JKI_lib_State_Machine.vi"("State(s) in (\"\")"=w338) -> ("States Out"=w337:string)  [unwired: 14 in]
      }
      frame "XY: Derivative" {
        # "Template Separator\n(You can make a copy of, or modify, this frame)"
        n137 = Unbundle By Name(w347) -> ("XY Data"=w348:cluster{"Intensity Data":dbl[], "Array":dbl[]}[])
        n138 = call-poly "Derivative.vi"("Type"="Interval Units", "error in (no error)"=w344, 9:"Derivative Type", 10:"Interval", "XY-data"=w348) -> ("error out"=w343:errorcluster, "Differential out"=→"Differential":cluster{"X-array":dbl[], "Y-array":dbl[]}, "XY-data out"=w345:cluster{"X-array":dbl[], "Y-array":dbl[]})  [unwired: 4 in]
        n139 = Bundle By Name(cluster=w347, "XY Data"=w345) -> (w346:T5)
        n140 = call <vilib>:"Add State(s) to Queue__JKI_lib_State_Machine.vi"("State(s) in (\"\")"=w350) -> ("States Out"=w349:string)  [unwired: 14 in]
      }
      frame "XY: Interpolate" {
        # "Template Separator\n(You can make a copy of, or modify, this frame)"
        n141 = Unbundle By Name(w356) -> ("XY Data"=w357:cluster{"Intensity Data":dbl[], "Array":dbl[]}[])
        n142 = call-poly "Interpolate.vi"("error in (no error)"=w353, "Configure"="Configure", "XY-data"=w357) -> ("error out"=w352:errorcluster, "Interpolated XY-data out"=w354:cluster{"X-array":dbl[], "Y-array":dbl[]}[])  [unwired: 7 in]
        n143 = Bundle By Name(cluster=w356, "XY Data"=w354) -> (w355:T5)
        n144 = call <vilib>:"Add State(s) to Queue__JKI_lib_State_Machine.vi"("State(s) in (\"\")"=w359) -> ("States Out"=w358:string)  [unwired: 14 in]
      }
      frame "XY: FFT Spectrum" {
        # "Template Separator\n(You can make a copy of, or modify, this frame)"
        n145 = Unbundle By Name(w365) -> ("XY Data"=w366:cluster{"Intensity Data":dbl[], "Array":dbl[]}[])
        n146 = call-poly "FFT Spectrum.vi"("error in (no error)"=w362, "XY-data"=w366) -> ("error out"=w361:errorcluster, "magnitude []"=w360:cluster{"f0":dbl, "df":dbl, "magnitude":dbl[]}[], "XY-data out"=w363:cluster{"X-array":dbl[], "Y-array":dbl[]}[])  [unwired: 6 in, 1 out]
        n147 = local write "FFT"(w360) -> ()
        n148 = Bundle By Name(cluster=w365, "XY Data"=w363) -> (w364:T5)
        n149 = call <vilib>:"Add State(s) to Queue__JKI_lib_State_Machine.vi"("State(s) in (\"\")"=w368) -> ("States Out"=w367:string)  [unwired: 14 in]
      }
      frame "XY: FFT Power Spectrum" {
        # "Template Separator\n(You can make a copy of, or modify, this frame)"
        n150 = Unbundle By Name(w374) -> ("XY Data"=w375:cluster{"Intensity Data":dbl[], "Array":dbl[]}[])
        n151 = call-poly "FFT Power Spectrum.vi"("error in (no error)"=w372, "XY-data"=w375) -> ("error out"=w371:errorcluster, "Power Spectrum"=→"FFT":cluster{"f0":dbl, "df":dbl, "magnitude":dbl[]}[], "XY-data out"=w370:cluster{"X-array":dbl[], "Y-array":dbl[]}[])  [unwired: 7 in]
        n152 = Bundle By Name(cluster=w374, "XY Data"=w370) -> (w373:T5)
        n153 = call <vilib>:"Add State(s) to Queue__JKI_lib_State_Machine.vi"("State(s) in (\"\")"=w377) -> ("States Out"=w376:string)  [unwired: 14 in]
      }
      frame "XY: Resample" {
        # "Template Separator\n(You can make a copy of, or modify, this frame)"
        n154 = Unbundle By Name(w382) -> ("XY Data"=w383:cluster{"Intensity Data":dbl[], "Array":dbl[]}[])
        n155 = call-poly "Resample.vi"("error in (no error)"=w379, "XY-data"=w383) -> ("error out"=w378:errorcluster, "Resampled XY-data out"=w380:cluster{"X-array":dbl[], "Y-array":dbl[]}[])  [unwired: 8 in]
        n156 = Bundle By Name(cluster=w382, "XY Data"=w380) -> (w381:T5)
        n157 = call <vilib>:"Add State(s) to Queue__JKI_lib_State_Machine.vi"("State(s) in (\"\")"=w385) -> ("States Out"=w384:string)  [unwired: 14 in]
      }
      frame "XY: Average" {
        # "Template Separator\n(You can make a copy of, or modify, this frame)"
        n158 = Unbundle By Name(w390) -> ("XY Data"=w391:cluster{"Intensity Data":dbl[], "Array":dbl[]}[])
        n159 = call "Average.vi"("error in (no error)"=w387, "XY-data"=w391) -> ("error out"=w386:errorcluster, "XY-data out"=w388:cluster{"X-array":dbl[], "Y-array":dbl[]}[])  [unwired: 7 in, 1 out]
        n160 = Bundle By Name(cluster=w390, "XY Data"=w388) -> (w389:T5)
        n161 = call <vilib>:"Add State(s) to Queue__JKI_lib_State_Machine.vi"("State(s) in (\"\")"=w393) -> ("States Out"=w392:string)  [unwired: 14 in]
      }
    }
  }
